vi "Get Map of Created Attributes.vi"(11 "Actor in":refnum<class "Actor.lvclass">) -> (2 "Map of Created Attributes":T1)   [LabVIEW 2020, in "jettl.lvlib" / "Actor.lvlib" / "Actor.lvclass"]
uses:
  Actor.lvclass
  Attributes/Attributes/Attributes.lvclass
  Map of Created Attributes.ctl
  Actor.lvlib
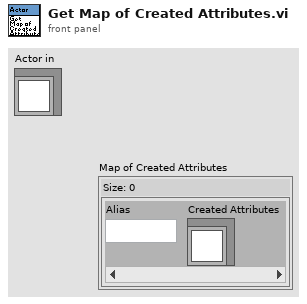
[diagram p1: front panel]
types:
  T1 = typedef "jettl.lvlib/Actor.lvlib/Map of Created Attributes.ctl" = map{string, refnum<class "Attributes.lvclass">}
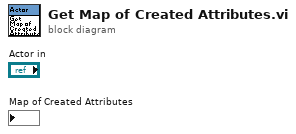
[diagram p0: block diagram]
diagram:
